vi "Create_Tree_Hierarchy.vi"() -> ()   [LabVIEW 2010]
uses:
  Anemometry/Anemometry Sub Vis/Controls/Global_mode.ctl
  Anemometry/Anemometry Sub Vis/Data_plotting_vis/Results_plotter_Global.vi
panel:
  out "Choose file":path
  in  "Tree Root":path
  in  "Header":string
  out "No Of input files":i32
  out "Index":i32
  in  "Folder":bool
  out "Precision":i32[](array[numeric])
  out "Filenames to append to":path[](array[path])
  out "Tree channel Indicies":i32[](array[numeric])
  out "Tolerances":dbl[](array[numeric]) format="%.2f"
  in  "Template":path=path "/G4_2_HD/Users/paulhayden/Sandia Internal Template"
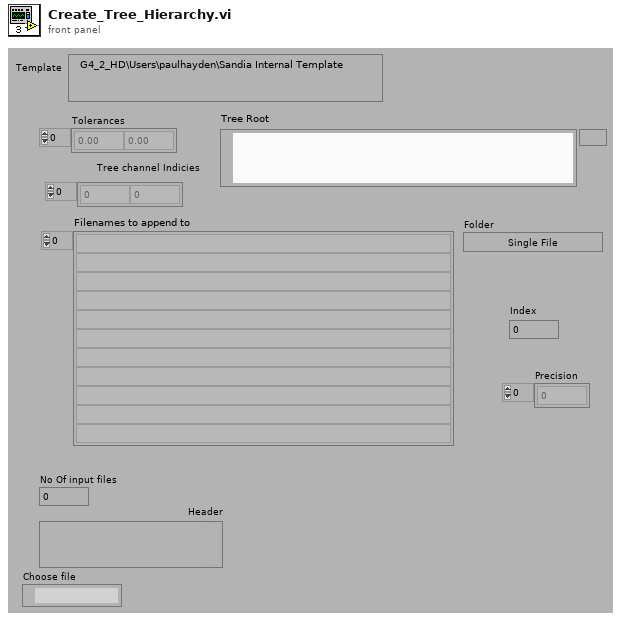
[diagram p1: front panel]
types:
  T1 = typedef "Global_mode.ctl" = enum16{"Read Global", "Load Global From File", "Write Global to File"}
  T2 = enum32{"existing file", "new file", "new or existing file", "existing dir", "new dir", "new or existing dir", "existing file (use LLBs)", "new file (use LLBs)", "new or existing file (use LLBs)", "new or existing file or directory (use LLBs)"}
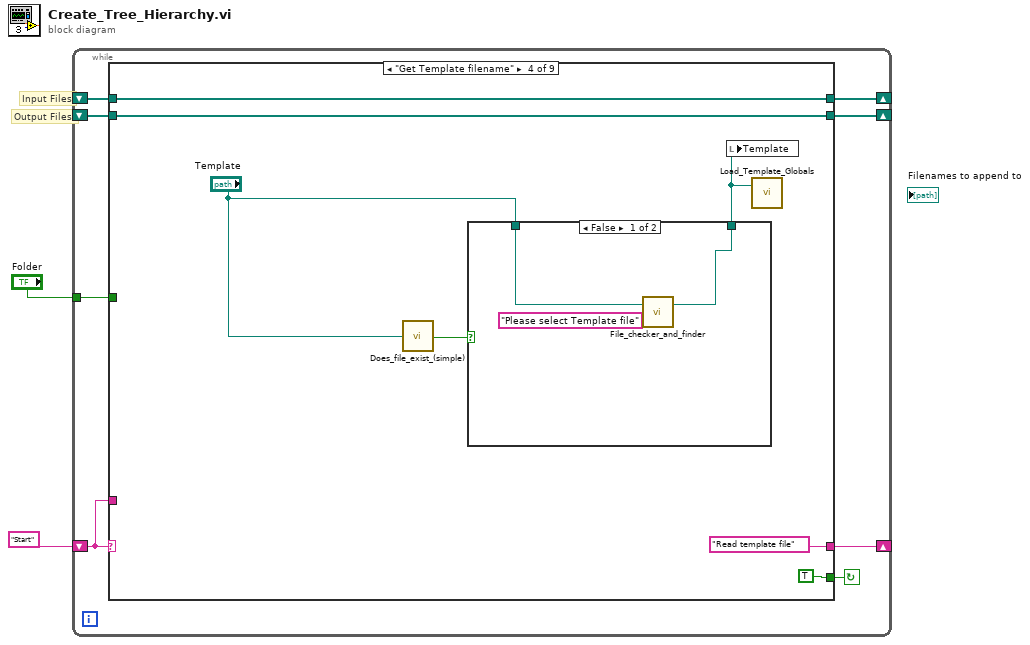
[diagram p0: block diagram]
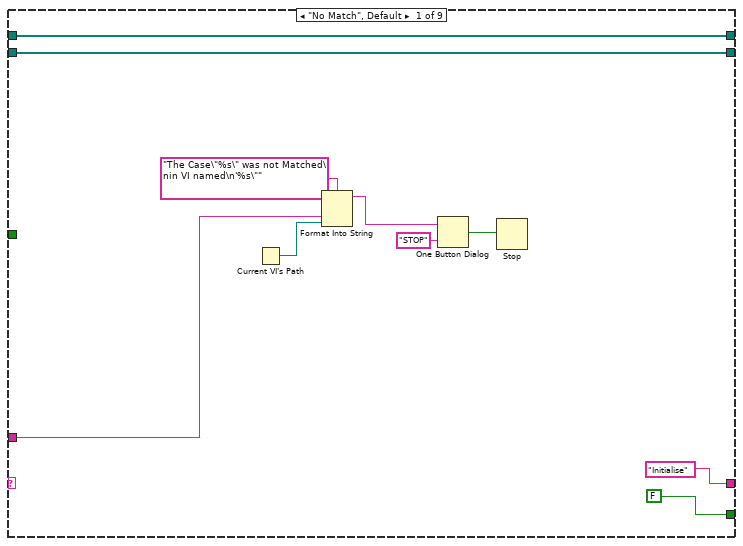
[diagram p2: hidden frame]
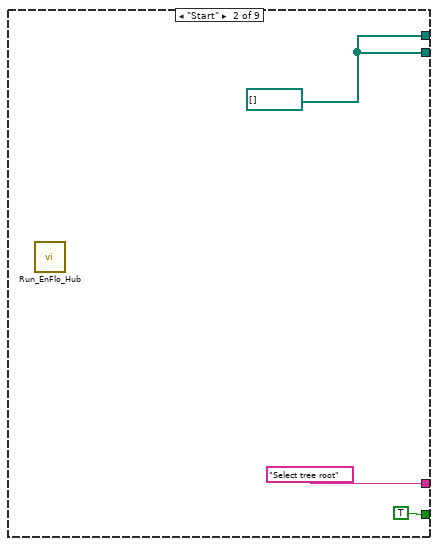
[diagram p3: hidden frame]
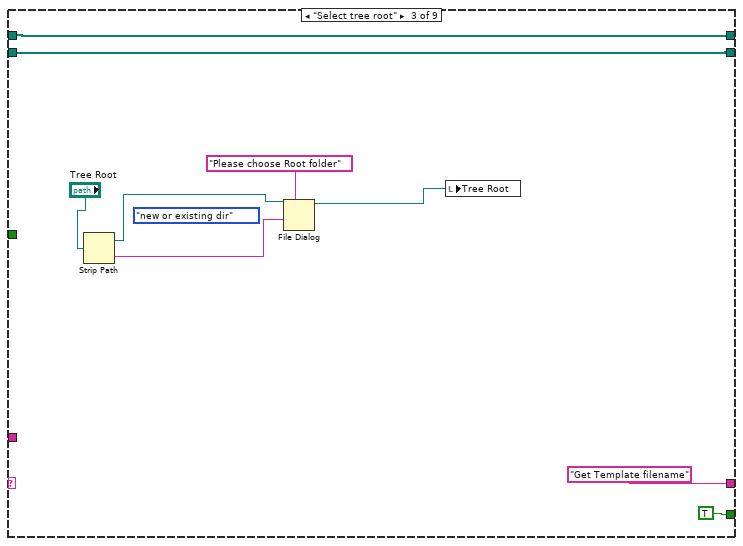
[diagram p4: hidden frame]
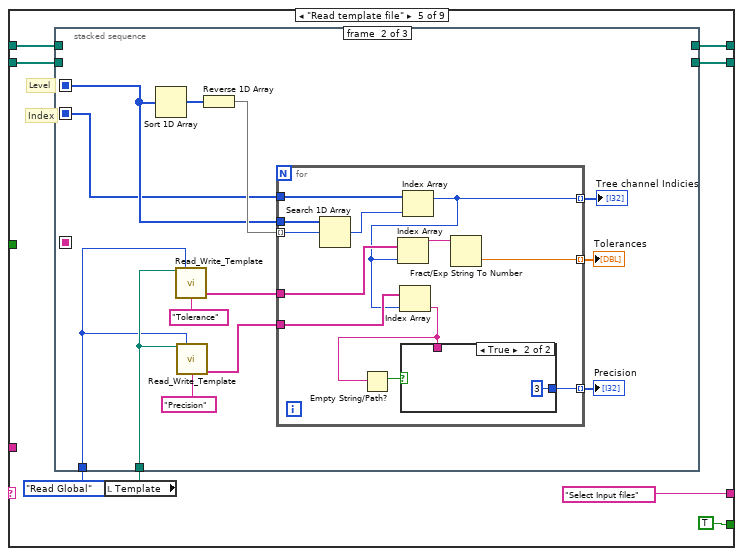
[diagram p6: hidden frame]
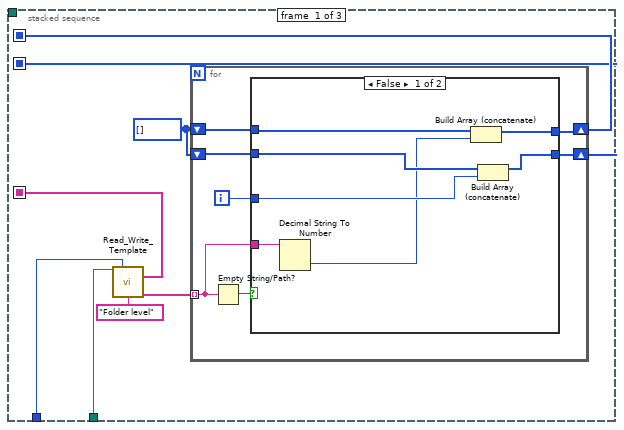
[diagram p7: hidden frame]
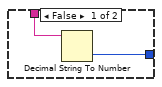
[diagram p9: hidden frame]
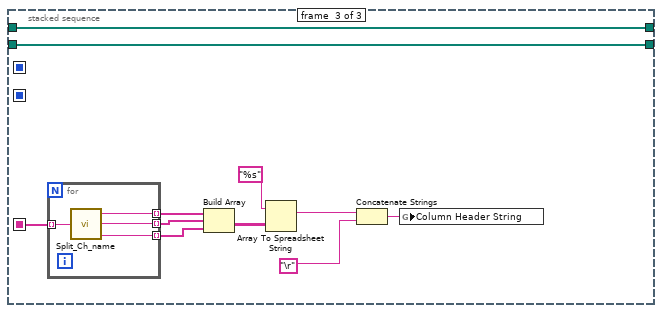
[diagram p10: hidden frame]
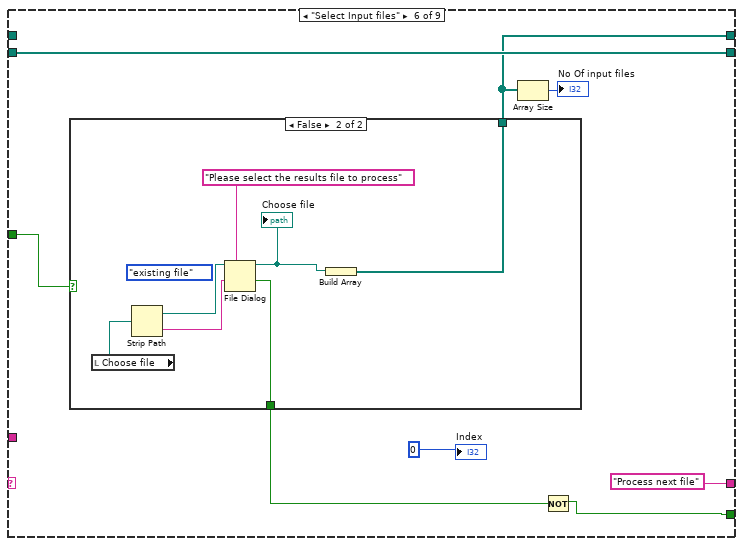
[diagram p11: hidden frame]
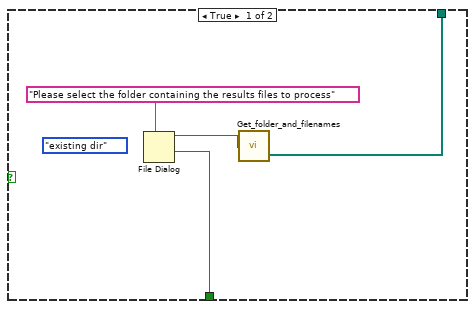
[diagram p12: hidden frame]
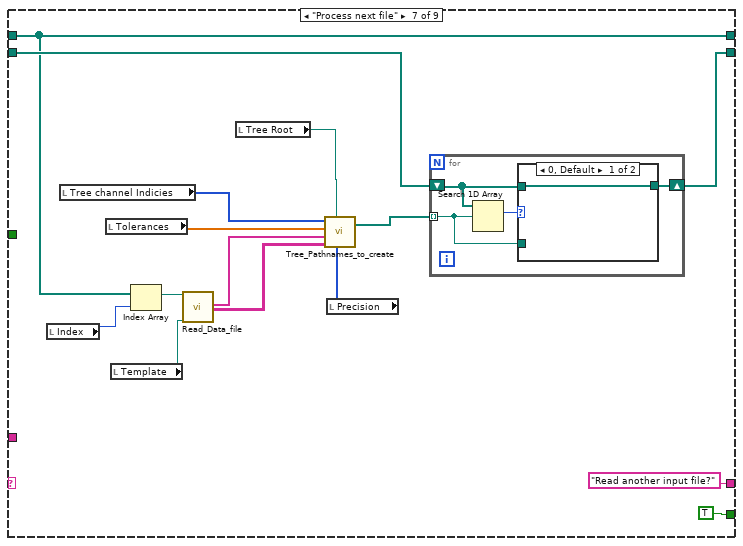
[diagram p13: hidden frame]
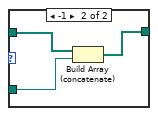
[diagram p14: hidden frame]
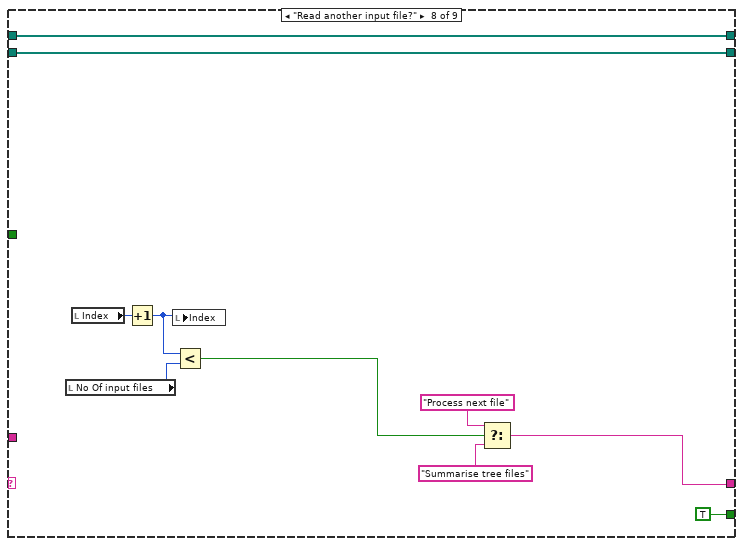
[diagram p15: hidden frame]
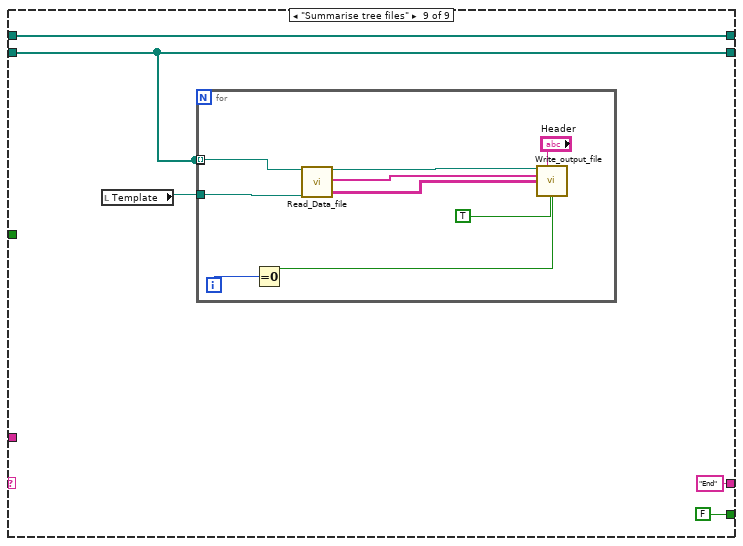
[diagram p16: hidden frame]
diagram:
  # "Output Files"
  # "Input Files"
  n1 = while {
    tunnel: "Folder" -> [w3]
    shift-left: _ -> [w4]
    shift-right: [w5] -> _
    shift-left: _ -> [w7]
    shift-right: [w6] -> _
    shift-left: "Start" -> [w8]
    shift-right: [w9] -> _
    stop <- w10 continue-if-true
    n2 = case shown="\"Get Template filename\"" w8 {
      tunnel: [FALSE TRUE TRUE TRUE TRUE w125 TRUE TRUE FALSE] -> w10
      tunnel: ["Initialise" "Select tree root" "Get Template filename" "Read template file" "Select Input files" "Process next file" "Read another input file?" w163 "End"] -> w9
      tunnel: w8 -> [w15 _ _ _ _ _ _ _ _]
      tunnel: w7 -> [w12 _ w29 w35 w47 _ w142 w170 w175]
      tunnel: [w12 w21 w29 w35 w46 w120 w142 w170 w175] -> w6
      tunnel: [w11 w21 w28 w34 w44 w124 w144 w169 w172] -> w5
      tunnel: w4 -> [w11 _ w28 w34 w45 w124 w146 w169 w172]
      tunnel: w3 -> [_ _ _ _ _ w123 _ _ _]
      frame "No Match", Default {
        n3 = Current VI's Path() -> (path=w14:path)
        n4 = Format Into String(format string="The Case\"%s\" was not Matched\nin VI named\n'%s\"" ("Format String"), w15, w14) -> (resulting string=w18:string)  [unwired: 2 in, 1 out]
        n5 = One Button Dialog(message=w18, button name ("OK")="STOP") -> (true=w16:bool)
        n6 = Stop(stop? (T)=w16) -> ()
      }
      frame "Start" {
        w21 = path[] [] ("Filenames to append to")
        n7 = call "Run_EnFlo_Hub.vi"() -> ()  [unwired: 8 in]
      }
      frame "Select tree root" {
        (unwired) T2."new or existing dir" ("select mode (2)")
        n8 = Strip Path(path="Tree Root") -> (stripped path=w25:path, name=w24:string)
        n9 = File Dialog(7:"Please choose Root folder" ("prompt"), 9:w24, 11:w25) -> (3:w27:path)  [unwired: 4 in, 3 out]
        n10 = local write "Tree Root"(w27) -> ()
      }
      frame "Get Template filename" {
        n11 = call "Does_file_exist_(simple).vi"("Pathname"="Template") -> ("exists?"=w36:bool)
        n12 = case shown="False" w36 {
          tunnel: "Template" -> [w41 w43]
          tunnel: [w40 w43] -> w33
          frame False {
            n13 = call "File_checker_and_finder.vi"("Promp if not found"="Please select Template file", "Filename In"=w41) -> ("Filename Out"=w40:path)  [unwired: 1 out]
          }
          frame True {
          }
        }
        n14 = local write "Template"(w33) -> ()
        n15 = call "Load_Template_Globals.vi"("Template-read"=w33) -> ()  [unwired: 1 in, 1 out]
      }
      frame "Read template file" {
        # "Index"
        # "Level"
        n16 = local read "Template"() -> (w49:path)
        n17 = stacked-sequence {
          seq-local: [w56 _ _] -> [_ w86 _]
          seq-local: [w55 _ _] -> [_ w84 _]
          seq-local: [w52 _ _] -> [_ _ w114]
          tunnel: w49 -> [w54 w81 _]
          tunnel: Global_mode."Read Global" ("Mode") -> [w53 w80 _]
          tunnel: w47 -> [_ _ w105]
          tunnel: [_ _ w105] -> w46
          tunnel: w45 -> [_ _ w104]
          tunnel: [_ _ w104] -> w44
          frame #0 {
            w57 = i32[] []
            n18 = call "Read_Write_Template.vi"("Template File"=w54, "Mode"=w53, "Data type"="Folder level") -> ("Template Ch Names Out"=w52:string[], "1D Info Out"=w58:string[])  [unwired: 6 in, 5 out]
            n19 = for {
              shift-right: [w63] -> w56
              shift-left: w57 -> [w64]
              shift-right: [w61] -> w55
              shift-left: w57 -> [w62]
              tunnel: w58 -> [w65] mode=indexing
              i -> [w60]
              n20 = Empty String/Path?(string/path=w65) -> (empty?=w66:bool)
              n21 = case shown="False" w66 {
                tunnel: w65 -> [w73 _]
                tunnel: w64 -> [w72 w75]
                tunnel: [w71 w75] -> w63
                tunnel: w62 -> [w70 w74]
                tunnel: [w69 w74] -> w61
                tunnel: w60 -> [w68 _]
                frame False {
                  n22 = Decimal String To Number(string=w73) -> (number=w67:i32)  [unwired: 2 in, 1 out]
                  n23 = Build Array (concatenate)(w72, w67) -> (w71:i32[])
                  n24 = Build Array (concatenate)(w70, w68) -> (w69:i32[])
                }
                frame True {
                }
              }
            }
          }
          frame #1 {
            n25 = Sort 1D Array(array=w86) -> (sorted array=w88:i32[])
            n26 = call "Read_Write_Template.vi"("Template File"=w81, "Mode"=w80, "Data type"="Tolerance") -> ("1D Info Out"=w78:string[])  [unwired: 6 in, 6 out]
            n27 = call "Read_Write_Template.vi"("Template File"=w81, "Mode"=w80, "Data type"="Precision") -> ("1D Info Out"=w77:string[])  [unwired: 6 in, 6 out]
            n28 = Reverse 1D Array(array=w88) -> (reversed array=w87:i32[])
            n29 = for {
              tunnel: w87 -> [w100] mode=indexing
              tunnel: w86 -> [w99]
              tunnel: w84 -> [w98]
              tunnel: [w92] -> w83 mode=indexing
              tunnel: [w97] -> w82 mode=indexing
              tunnel: w78 -> [w95]
              tunnel: w77 -> [w93]
              tunnel: [w89] -> w76 mode=indexing
              n30 = Search 1D Array(1D array=w99, element=w100) -> (index of element=w96:i32)  [unwired: 1 in]
              n31 = Index Array(array=w98, index=w96) -> (element=w92:i32)
              n32 = Index Array(array=w95, index=w92) -> (element=w94:string)
              n33 = Index Array(array=w93, index=w92) -> (element=w90:string)
              n34 = Empty String/Path?(string/path=w90) -> (empty?=w91:bool)
              n35 = case shown="True" w91 {
                tunnel: w90 -> [w102 _]
                tunnel: [w101 3] -> w89
                frame False {
                  n36 = Decimal String To Number(string=w102) -> (number=w101:i32)  [unwired: 2 in, 1 out]
                }
                frame True {
                }
              }
              n37 = Fract/Exp String To Number(string=w94) -> (number=w97:dbl)  [unwired: 3 in, 1 out]
            }
            "Tolerances" <- w82
            "Tree channel Indicies" <- w83
            "Precision" <- w76
          }
          frame #2 {
            n38 = for {
              tunnel: w114 -> [w118] mode=indexing
              tunnel: [w117] -> w113 mode=indexing
              tunnel: [w116] -> w112 mode=indexing
              tunnel: [w115] -> w111 mode=indexing
              n39 = call "Split_Ch_name.vi"("Ch name"=w118) -> ("Top level"=w117:string, "Middle"=w116:string, "Low level"=w115:string)
            }
            n40 = Build Array(w113, w112, w111) -> (w110:string[][])
            n41 = Array To Spreadsheet String(array=w110, 3:"%s" ("format string")) -> (spreadsheet string=w108:string)  [unwired: 1 in]
            n42 = Concatenate Strings(w108, "\r") -> (w106:string)
            n43 = global write "Results_plotter_Global.vi" "Column Header String"(w106) -> ()
          }
        }
      }
      frame "Select Input files" {
        n44 = case shown="False" w123 {
          tunnel: [w129 w136] -> w120
          tunnel: [w128 w135] -> w122
          frame True {
            (unwired) T2."existing dir" ("select mode (2)")
            n45 = File Dialog(7:"Please select the folder containing the results files to process" ("prompt")) -> (1:w128:bool, 3:w130:path)  [unwired: 6 in, 2 out]
            n46 = call "Get_folder_and_filenames.vi"("file path (dialog if empty)"=w130) -> ("Files"=w129:path[])  [unwired: 1 out]
          }
          frame False {
            (unwired) T2."existing file" ("select mode (2)")
            n47 = local read "Choose file"() -> (w131:path)
            n48 = Strip Path(path=w131) -> (stripped path=w133:path, name=w132:string)
            n49 = File Dialog(7:"Please select the results file to process" ("prompt"), 9:w132, 11:w133) -> (1:w135:bool, 3:w137:path)  [unwired: 4 in, 2 out]
            "Choose file" <- w137
            n50 = Build Array(w137) -> (w136:path[])
          }
        }
        n51 = Array Size(array=w120) -> (size(s)=→"No Of input files":i32)
        n52 = Not(x=w122) -> (.not. x?=w125:bool)
        "Index" <- 0
      }
      frame "Process next file" {
        n53 = local read "Index"() -> (w143:i32)
        n54 = local read "Tree channel Indicies"() -> (w149:i32[])
        n55 = local read "Tolerances"() -> (w150:dbl[])
        n56 = local read "Template"() -> (w141:path)
        n57 = Index Array(array=w142, index=w143) -> (element=w148:path)
        n58 = call "Read_Data_file.vi"("Results file"=w148, "Template File"=w141) -> ("Ch names Out"=w140:string[], "Channel Values Out"=w139:string[][])  [unwired: 8 in, 8 out]
        n59 = local read "Tree Root"() -> (w138:path)
        n60 = local read "Precision"() -> (w147:i32[])
        n61 = call "Tree_Pathnames_to_create.vi"("Precision"=w147, "Tree Root"=w138, "Channel Values In"=w139, "Ch names In"=w140, "Tree channel Tolerances"=w150, "Tree channel Indicies"=w149) -> ("Filenames to append to"=w145:path[])  [unwired: 1 in]
        n62 = for {
          shift-right: [w153] -> w144
          shift-left: w146 -> [w155]
          tunnel: w145 -> [w154] mode=indexing
          n63 = Search 1D Array(1D array=w155, element=w154) -> (index of element=w156:i32)  [unwired: 1 in]
          n64 = case shown="0, Default" w156 {
            tunnel: w155 -> [w157 w160]
            tunnel: w154 -> [_ w159]
            tunnel: [w157 w158] -> w153
            frame 0, Default {
            }
            frame -1 {
              n65 = Build Array (concatenate)(w160, w159) -> (w158:path[])
            }
          }
        }
      }
      frame "Read another input file?" {
        n66 = local read "No Of input files"() -> (w166:i32)
        n67 = local read "Index"() -> (w168:i32)
        n68 = Increment(x=w168) -> (x+1=w167:i32)
        n69 = local write "Index"(w167) -> ()
        n70 = Less?(x=w167, y=w166) -> (x < y?=w162:bool)
        n71 = Select(t="Process next file", s=w162, f="Summarise tree files") -> (s? t:f=w163:string)
      }
      frame "Summarise tree files" {
        n72 = local read "Template"() -> (w171:path)
        n73 = for {
          tunnel: w172 -> [_] mode=indexing
          tunnel: w172 -> [w182] mode=indexing
          tunnel: w171 -> [w179]
          i -> [w177]
          n74 = Equal To 0?(x=w177) -> (x = 0?=w176:bool)
          n75 = call "Read_Data_file.vi"("Results file"=w182, "Template File"=w179) -> ("Results file Out"=w180:path, "Ch names Out"=w181:string[], "Channel Values Out"=w178:string[][])  [unwired: 8 in, 7 out]
          n76 = call "Write_output_file.vi"("Output filename"=w180, "Header"="Header", "Channel Names"=w181, "Data"=w178, "Save Plotted rows only?"=TRUE ("Overwrite File"), "Summarise mode"=w176) -> ()  [unwired: 9 in, 1 out]
        }
      }
    }
  }
